vi "Soft Stops.vi"(0 "Motor In":dbl=0.04, 1 "Disable Softstops":bool, 2 "Disable Motor":bool, 3 "correlation":bool=TRUE, 5 "Sense":dbl, 9 "Lo Limit":dbl=-10.0, 11 "Hi Limit":dbl=35.0, 12 "Speed near Limit":dbl=0.02, 13 "Near Limit":dbl=1.0, 14 "Motor Coerce":dbl=1.0) -> (4 "Motor Out":dbl, 10 "At Lo":bool, 15 "At Hi":bool)   [LabVIEW 2015]
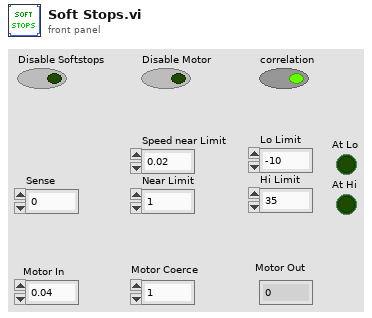
[diagram p1: front panel]
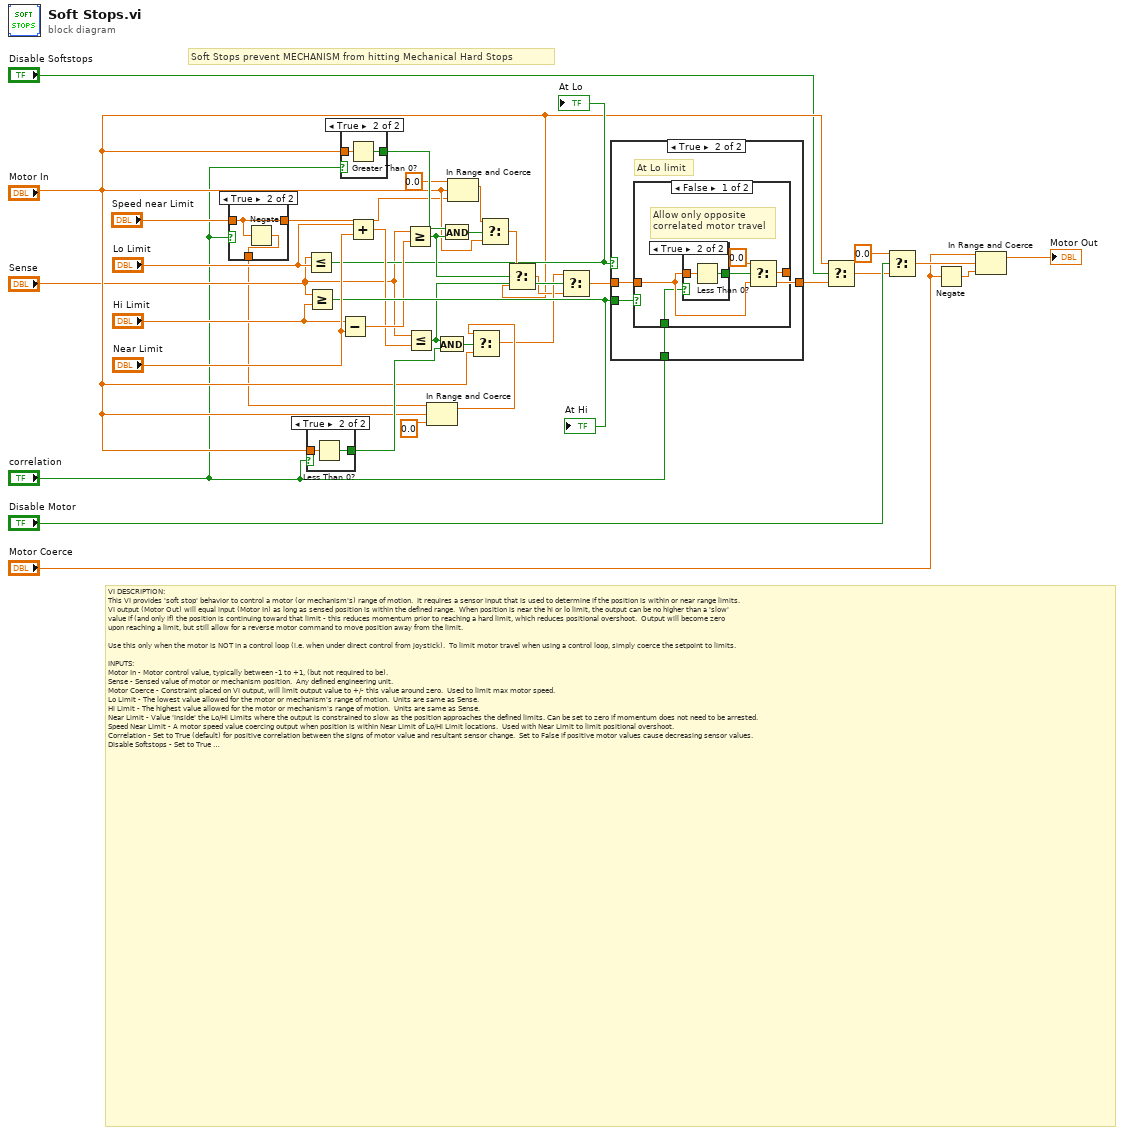
[diagram p0: block diagram]
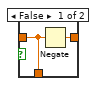
[diagram p2: hidden frame]
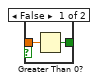
[diagram p3: hidden frame]
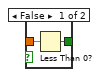
[diagram p4: hidden frame]
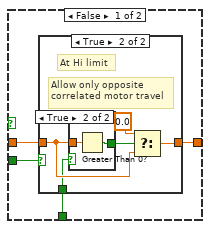
[diagram p5: hidden frame]
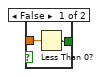
[diagram p7: hidden frame]
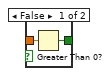
[diagram p8: hidden frame]
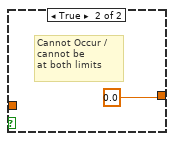
[diagram p9: hidden frame]
diagram:
  # "VI DESCRIPTION:\nThis VI provides 'soft stop' behavior to control a motor (or mechanism's) range of motion.  It requires a sensor input that is used to determine if the position is within or near range limits.\nVI output (Motor Out) will equal input (Motor In) as long as sensed position is within the defined range.  When position is near the hi or lo limit, the output can be no higher than a 'slow'\nvalue if (and only if) the position is continuing toward that limit - this reduces momentum prior to reaching a hard limit, which reduces positional overshoot.  Output will become zero \nupon reaching a limit, but still allow for a reverse motor command to move position away from the limit.\n\nUse this only when the motor is NOT in a control loop (i.e. when under direct control from joystick).  To limit motor travel when using a control loop, simply coerce the setpoint to limits.\n\nINPUTS:\nMotor In - Motor control value, typically between -1 to +1, (but not required to be).\nSense - Sensed value of motor or mechanism position.  Any defined engineering unit.\nMotor Coerce - Constraint placed on VI output, will limit output value to +/- this value around zero.  Used to limit max motor speed.\nLo Limit - The lowest value allowed for the motor or mechanism's range of motion.  Units are same as Sense.\nHi Limit - The highest value allowed for the motor or mechanism's range of motion.  Units are same as Sense.\nNear Limit - Value 'inside' the Lo/Hi Limits where the output is constrained to slow as the position approaches the defined limits. Can be set to zero if momentum does not need to be arrested.\nSpeed Near Limit - A motor speed value coercing output when position is within Near Limit of Lo/Hi Limit locations.  Used with Near Limit to limit positional overshoot.\nCorrelation - Set to True (default) for positive correlation between the signs of motor value and resultant sensor change.  Set to False if positive motor values cause decreasing sensor values.\nDisable Softstops - Set to True to over ride the softstop behavor and pass Motor In directly to Motor Out.\nDisable Motor - Set to True to send value zero to Motor Output.  If both Disables are selected, Disable Motor takes precedence over Disable Softstops.\n\nOUTPUTS:\nMotor Out - Motor control value modified by VI behavior.\nAt Lo - Boolean indicating status of sensed position, True if equal or lower than Lo Limit.\nAt Hi - Boolean indicating status of sensed position, True if equal or higher than Hi Limit.\n\nIMPLEMENTATION:\nDo not use in a control loop, use setpoint coercion instead for this situation.  For direct motor control:\nDetermine the correlation of the mechanical arrangement; if positive motor values cause increasing sensor values, set Correlation to True.\nDetermine the physical limits of the mechanism and set Lo and Hi Limits just short of these limits, by an amount that will accomodate any small overshoot that might remain after tuning.\nTo limit positional overshoot, create a region just inside each limit to slow the motor by setting Near Limit.\nSet Speed Near Limit to a value slow enough to bring the mechanism to a stop prior to reaching physical limits.\nSet Motor Coerce to the maximum speed that the mechanism is allowed to travel.\nExperimentally determine values that minimize the Near Limit region and maximize Speed Near Limit, without striking the mechanism's physical limits when approaching at full speed.\n\n\nFIRST Team 836, RoboBees"
  # "Soft Stops prevent MECHANISM from hitting Mechanical Hard Stops"
  n1 = case shown="True" "correlation" {
    tunnel: "Speed near Limit" -> [w37 w39]
    tunnel: [w38 w39] -> w6
    tunnel: [w37 w40] -> w3
    frame False {
      n2 = Negate(x=w37) -> (-x=w38:dbl)
    }
    frame True {
      n3 = Negate(x=w39) -> (-x=w40:dbl)
    }
  }
  n4 = Less Or Equal?(x="Sense", y="Lo Limit") -> (x <= y?=w11:bool)
  "At Lo" <- w11
  n5 = Greater Or Equal?(x="Sense", y="Hi Limit") -> (x >= y?=w34:bool)
  "At Hi" <- w34
  n6 = case shown="True" "correlation" {
    tunnel: [w42 w43] -> w24
    tunnel: "Motor In" -> [w41 w44]
    frame False {
      n7 = Greater Than 0?(x=w41) -> (x > 0?=w42:bool)
    }
    frame True {
      n8 = Less Than 0?(x=w44) -> (x < 0?=w43:bool)
    }
  }
  n9 = Subtract(x="Hi Limit", y="Near Limit") -> (x-y=w32:dbl)
  n10 = case shown="True" "correlation" {
    tunnel: [w46 w47] -> w29
    tunnel: "Motor In" -> [w45 w48]
    frame False {
      n11 = Less Than 0?(x=w45) -> (x < 0?=w46:bool)
    }
    frame True {
      n12 = Greater Than 0?(x=w48) -> (x > 0?=w47:bool)
    }
  }
  n13 = Add(x="Lo Limit", y="Near Limit") -> (x+y=w31:dbl)
  n14 = Greater Or Equal?(x="Sense", y=w32) -> (x >= y?=w22:bool)
  n15 = Less Or Equal?(x="Sense", y=w31) -> (x <= y?=w20:bool)
  n16 = In Range and Coerce(upper limit=w3, x="Motor In", lower limit=0.0 ("upper limit")) -> (coerced(x)=w23:dbl)  [unwired: 1 out]
  n17 = And(x=w20, y=w24) -> (x .and. y?=w26:bool)
  n18 = And(x=w29, y=w22) -> (x .and. y?=w30:bool)
  n19 = In Range and Coerce(upper limit=0.0, x="Motor In", lower limit=w6) -> (coerced(x)=w28:dbl)  [unwired: 1 out]
  n20 = Select(t=w23, s=w26, f="Motor In") -> (s? t:f=w19:dbl)
  n21 = Select(t=w28, s=w30, f="Motor In") -> (s? t:f=w21:dbl)
  n22 = Select(t=w21, s=w22, f="Motor In") -> (s? t:f=w18:dbl)
  n23 = Select(t=w19, s=w20, f=w18) -> (s? t:f=w17:dbl)
  n24 = case shown="True" w11 {
    tunnel: [w50 w65] -> w33
    tunnel: w17 -> [w52 w66]
    tunnel: w34 -> [w51 w64]
    tunnel: "correlation" -> [w49 w63]
    frame False {
      n25 = case shown="True" w51 {
        tunnel: w52 -> [w53 w56]
        tunnel: [w53 w55] -> w50
        tunnel: w49 -> [_ w54]
        frame False {
          # "At neither limit"
        }
        frame True {
          # "Allow only opposite\ncorrelated motor travel"
          # "At Hi limit"
          n26 = case shown="True" w54 {
            tunnel: [w60 w61] -> w58
            tunnel: w56 -> [w59 w62]
            frame False {
              n27 = Less Than 0?(x=w59) -> (x < 0?=w60:bool)
            }
            frame True {
              n28 = Greater Than 0?(x=w62) -> (x > 0?=w61:bool)
            }
          }
          n29 = Select(t=0.0, s=w58, f=w56) -> (s? t:f=w55:dbl)
        }
      }
    }
    frame True {
      # "At Lo limit"
      n30 = case shown="False" w64 {
        tunnel: w66 -> [w68 _]
        tunnel: [w69 0.0 ("Turret Yaw Control")] -> w65
        tunnel: w63 -> [w67 _]
        frame False {
          # "Allow only opposite\ncorrelated motor travel"
          n31 = case shown="True" w67 {
            tunnel: [w73 w74] -> w71
            tunnel: w68 -> [w72 w75]
            frame False {
              n32 = Greater Than 0?(x=w72) -> (x > 0?=w73:bool)
            }
            frame True {
              n33 = Less Than 0?(x=w75) -> (x < 0?=w74:bool)
            }
          }
          n34 = Select(t=0.0, s=w71, f=w68) -> (s? t:f=w69:dbl)
        }
        frame True {
          # "Cannot Occur / \ncannot be \nat both limits"
        }
      }
    }
  }
  n35 = Select(t="Motor In", s="Disable Softstops", f=w33) -> (s? t:f=w5:dbl)
  n36 = Select(t=0.0, s="Disable Motor", f=w5) -> (s? t:f=w15:dbl)
  n37 = Negate(x="Motor Coerce") -> (-x=w14:dbl)
  n38 = In Range and Coerce(upper limit="Motor Coerce", x=w15, lower limit=w14) -> (coerced(x)=→"Motor Out":dbl)  [unwired: 1 out]
